vi "DoubleAxisHomeFunction.vi"(10 "Axis 2":string, 11 "Axis 1":string) -> (2 "Y Position":string, 3 "X Position":string)   [LabVIEW 2016]
uses:
  Examples/Motion/EnableMultiple.vi
  Examples/Motion/HomeMultiple.vi
  Examples/Motion/DisableMultiple.vi
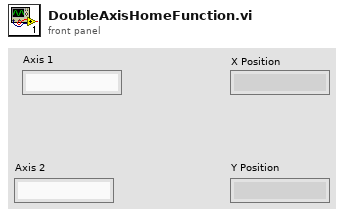
[diagram p1: front panel]
types:
  T1 = typedef "ControllerDiagPacket.ctl" = cluster{"Number of Diag Packets":i32, "Axes":T2[], "error":errorcluster}
  T2 = typedef "AxisDiagPacket.ctl" = cluster{"Axis Name":string, "Analog Input 0":dbl, "Analog Input 1":dbl, "Axis Fault (num)":i32, "Axis Fault (str)":string, "Axis Fault (bits)":cluster{"AmplifierFault":bool, "AmplifierTemperatureFault":bool, "CcwEndOfTravelLimitFault":bool, "CcwSoftwareLimitFault":bool, "CommunicationLostFault":bool, "CwEndOfTravelLimitFault":bool, "CwSoftwareLimitFault":bool, "EmergencyStopFault":bool, "EncoderFault":bool, "ExternalFault":bool, "FeedbackScalingFault":bool, "GantryMisalignFault ":bool, "HallSensorFault":bool, "InPositionTimeoutFault":bool, "MarkerSearchFault":bool, "MaxVelocityCommandFault":bool, "MissedInterruptFault":bool, "MotorTemperatureFault":bool, "None":bool, "OverCurrentFault":bool, "PositionErrorFault":bool, "PositionFeedbackFault":bool, "PowerSupplyFault":bool, "ProbeInputFault":bool, "SafeZoneFault":bool, "VelocityErrorFault":bool, "VelocityFeedbackFault":bool, "VoltageClampFault":bool}, "Axis Status (num)":i32, "Axis Status (str)":string, "Axis Status (bits)":cluster{"BacklashActive":bool, "CalibrationEnabled1D":bool, "CalibrationEnabled2D":bool, "CommandValid":bool, "DriveAbortPending":bool, "DrivePending":bool, "Enabling":bool, "GainMappingEnabled":bool, "GantryAligned":bool, "GantryRealigning":bool, "Homed":bool, "Homing":bool, "IFOVEnabled":bool, "JogGenerating":bool, "Jogging":bool, "JoystickControl":bool, "MasterSlaveControl":bool, "MotionBlocked":bool, "MotionClamped":bool, "MoveDone":bool, "None":bool, "NotVirtual":bool, "Profiling":bool, "Stability0":bool, "Stability1":bool, "TrajectoryFiltering":bool, "WaitDone":bool}, "Current Command":sgl, "Current Error":sgl, "Current Feedback":sgl, "Digital Inputs":i32, "Digital Outputs":i32, "Drive Status":i32, "Drive Status (str)":string, "Drive Status (bits)":cluster{"AccelerationPhase":bool, "AutofocusActive":bool, "BrakeOutput":bool, "CcwEndOfTravelLimitInput":bool, "CosineEncoderError":bool, "CurrentClamp":bool, "CwEndOfTravelLimitInput":bool, "DecelerationPhase":bool, "DualLoopActive":bool, "EmergencyStopInput":bool, "Enabled":bool, "EncoderClipping":bool, "GalvoCalibrationEnabled":bool, "GalvoPowerCorrection":bool, "HallAInput":bool, "HallBInput":bool, "HallCInput":bool, "HighResolutionMode":bool, "HomeLimitInput":bool, "InPosition":bool, "InPosition2":bool, "MarkerInput":bool, "MarkerLatch":bool, "MoveActive":bool, "NoMotorSupply":bool, "None":bool, "PowerLimiting":bool, "ProgrammingFlash":bool, "ProgrammingMXH":bool, "PSOHaltLatch":bool, "ServoControl":bool, "SineEncoderError":bool}, "Position Feedback Auxiliary":dbl, "Position Command":dbl, "Position Error":dbl, "Position Feedback":dbl, "Program Position Command":dbl, "Program Position Error":dbl, "Program Position Feedback":dbl, "Velocity Command":dbl, "Velocity Error":dbl, "Velocity Feedback":dbl}
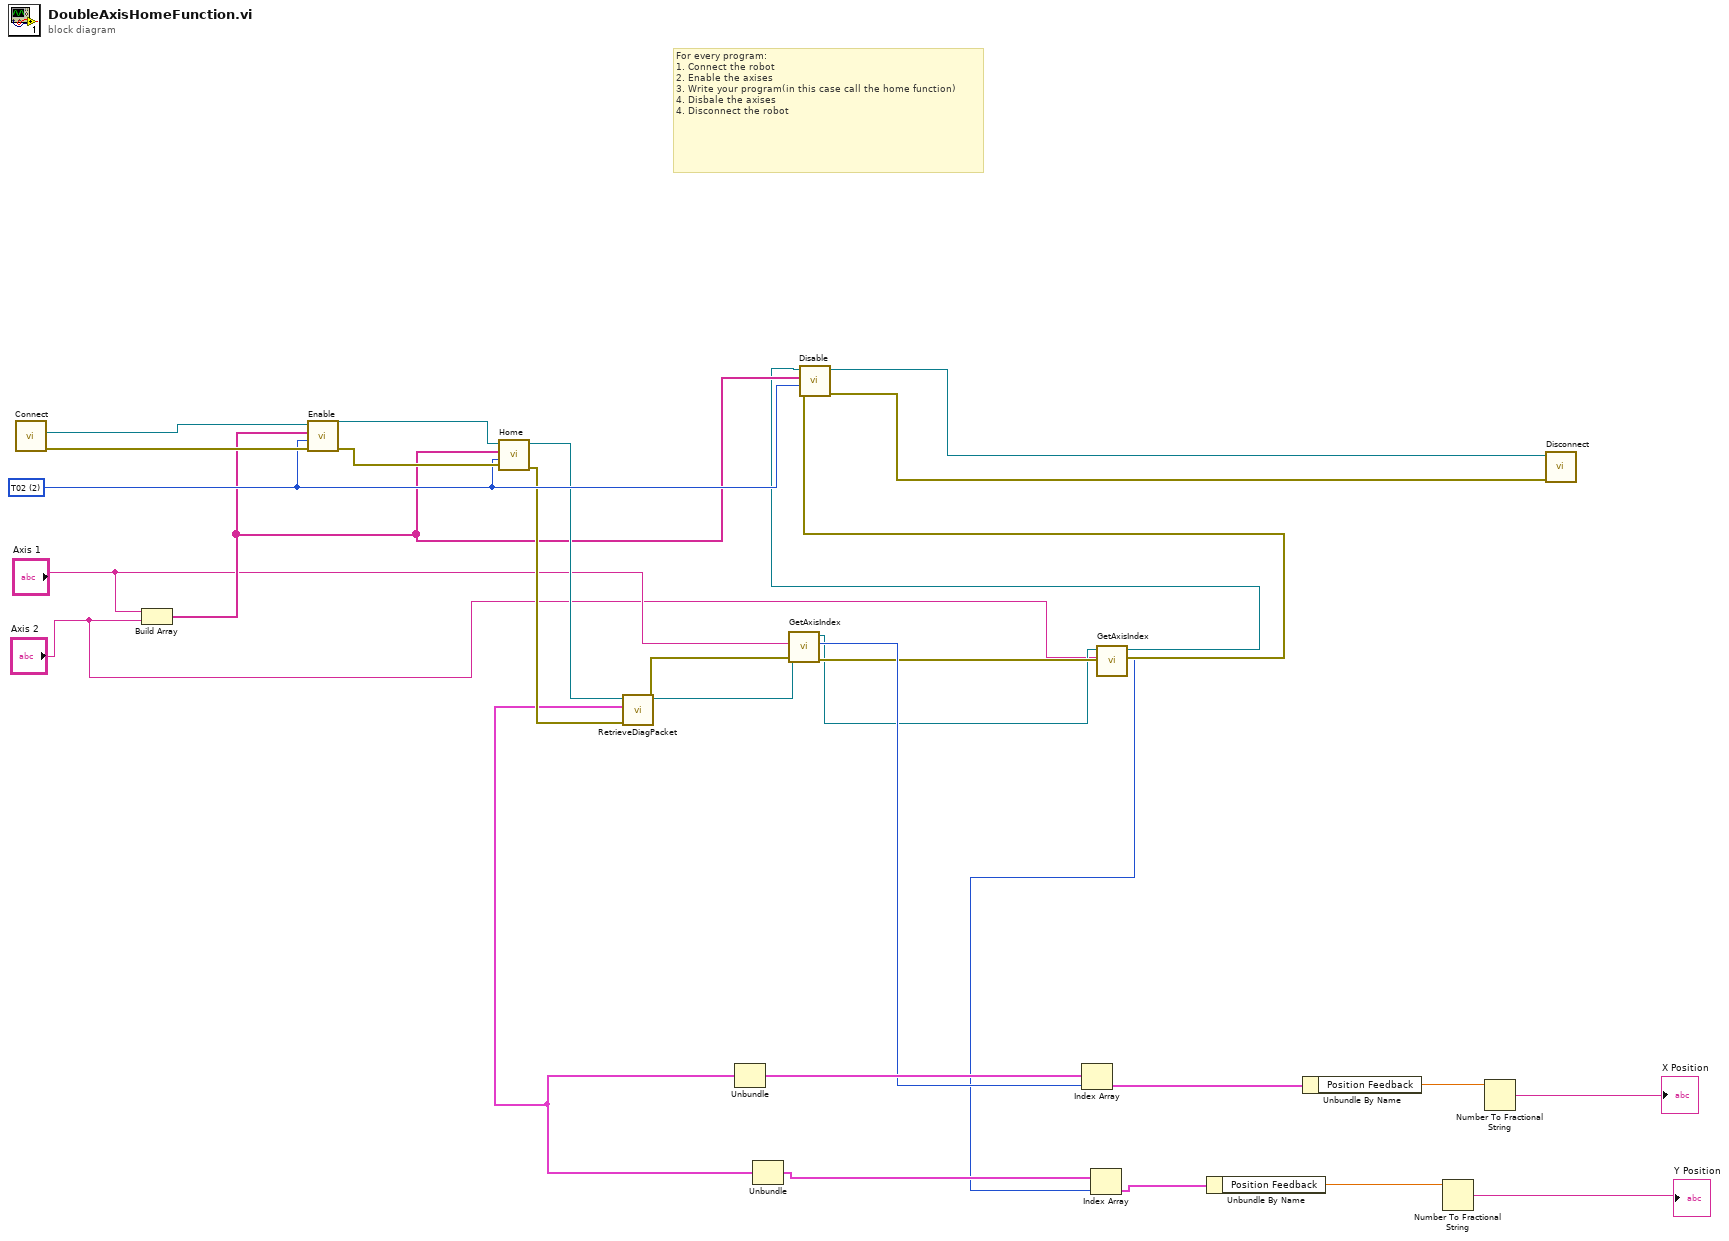
[diagram p0: block diagram]
diagram:
  w23 = 2 items=["TLibrary", "T01", "T02", "T03", "T04", "T05", "T06", "T07", "T08", "T09", "T10", "T11", "T12", "T13", "T14", "T15", "T16", "T17", "T18", "T19", "T20", "T21", "T22", "T23", "T24", "T25", "T26", "T27", "T28", "T29", "T30", "T31"] ("taskId")
  # "For every program:\n1. Connect the robot\n2. Enable the axises\n3. Write your program(in this case call the home function)\n4. Disbale the axises\n4. Disconnect the robot"
  n1 = call "Connect.vi"() -> ("error out"=w26:errorcluster, "controller"=w29:refnum<k24>)  [unwired: 10 in]
  n2 = Build Array("Axis 1", "Axis 2") -> (w13:string[])
  n3 = call-poly "Enable.vi"("error in (no error)"=w26, "taskId"=w23, "axis names"=w13, "controller in"=w29) -> ("error out"=w25:errorcluster, "controller out"=w28:refnum<k24>)  [unwired: 6 in]
  n4 = call-poly "Home.vi"("error in (no error)"=w25, "taskId"=w23, "axis names"=w13, "controller in"=w28) -> ("error out"=w20:errorcluster, "controller out"=w22:refnum<k24>)  [unwired: 6 in]
  n5 = call "RetrieveDiagPacket.vi"("error in (no error)"=w20, "Controller In"=w22) -> ("error out"=w19:errorcluster, "ControllerDiagPacket"=w7:T1, "Controller Out"=w21:refnum<k24>)  [unwired: 7 in]
  n6 = Unbundle "Unbundle"(w7) -> ("Axes"=w18:T2[])  [unwired: 2 out]
  n7 = Unbundle "Unbundle"(w7) -> ("Axes"=w6:T2[])  [unwired: 2 out]
  n8 = call "GetAxisIndex.vi"("error in (no error)"=w19, "axis name"="Axis 1", "controller in"=w21) -> ("error out"=w11:errorcluster, "axis index"=w17:i32, "controller out"=w9:refnum<k24>)  [unwired: 6 in]
  n9 = Index Array "Index Array"(array=w18, index=w17) -> (element=w16:T2)
  n10 = call "GetAxisIndex.vi"("error in (no error)"=w11, "axis name"="Axis 2", "controller in"=w9) -> ("error out"=w10:errorcluster, "axis index"=w5:i32, "controller out"=w8:refnum<k24>)  [unwired: 6 in]
  n11 = call-poly "Disable.vi"("error in (no error)"=w10, "taskId"=w23, "axis names"=w13, "controller in"=w8) -> ("error out"=w24:errorcluster, "controller out"=w27:refnum<k24>)  [unwired: 6 in]
  n12 = Index Array "Index Array"(array=w6, index=w5) -> (element=w3:T2)
  n13 = Unbundle By Name "Unbundle By Name"(w3) -> ("Position Feedback"=w4:dbl)
  n14 = Unbundle By Name "Unbundle By Name"(w16) -> ("Position Feedback"=w15:dbl)
  n15 = Number To Fractional String(number=w4) -> (F-format string=→"Y Position":string)  [unwired: 3 in]
  n16 = Number To Fractional String(number=w15) -> (F-format string=→"X Position":string)  [unwired: 3 in]
  n17 = call "Disconnect.vi"("error in (no error)"=w24, "controller"=w27) -> ()  [unwired: 9 in, 1 out]
